vi "Read DeviceSettings.vi"(8 "error in (no error)":errorcluster, 11 "NhRegenGridSim in":refnum<class "NHRGridSim.lvclass">) -> (0 "error out":errorcluster, 2 "DeviceSettings":T1 {"Modules"."Phase (0: All)" items=["All", "A Phase", "B Phase", "C Phase"]; "Modules"."Mode" items=["3-Phase AC", "AC", "DC", "AC - AC - AC", "DC - DC - DC", "2-Phase AC - AC", "2-Phase AC - DC", "AC - AC", "AC - DC", "AC - AC - DC", "AC - DC - DC", "DC - AC", "DC - DC", "AC - DC - AC", "DC - AC - AC", "DC - AC - DC"]}, 3 "NhRegenGridSim out":refnum<class "NHRGridSim.lvclass">)   [LabVIEW 2018, in "AcPwrPlugins.lvlib" / "NHRGridSim.lvclass"]
uses:
  NHRGridSim.lvclass
  TypeDefs/Device(s)Settings_old.ctl
  TypeDefs/Modules.ctl
  NHRGridSim.lvclass/NHRGridSim.ctl
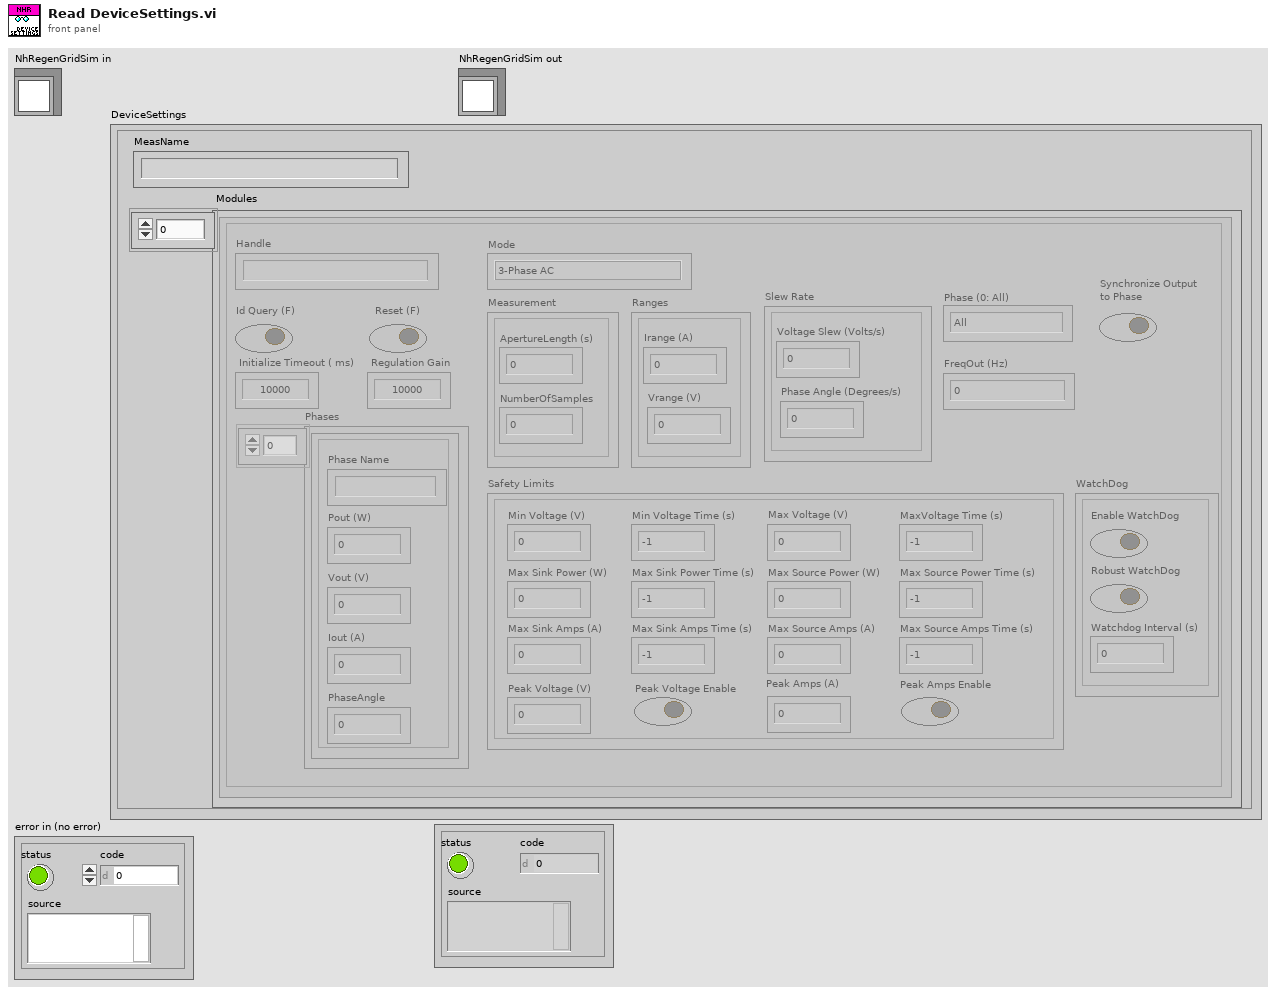
[diagram p1: front panel]
types:
  T1 = typedef "Device(s)Settings_old.ctl" = cluster{"MeasName":string, "Modules":T2}
  T2 = typedef "AcPwrPlugins.lvlib/NHRGridSim.lvclass/Modules.ctl" = cluster{"Measurement":cluster{"ApertureLength (s)":dbl, "NumberOfSamples":u32}, "Ranges":cluster{"Irange (A)":dbl, "Vrange (V)":dbl}, "Mode":u8, "Handle":string, "FreqOut (Hz)":dbl, "Connected":bool, "btnIdQuery":bool, "btnReset":bool, "Initialize Timeout ( ms)":u32, "Phase (0: All)":i32, "WatchDog":cluster{"Enable WatchDog":bool, "Robust WatchDog":bool, "Watchdog Interval (s)":dbl}, "Safety Limits":cluster{"Min Voltage (V)":dbl, "Min Voltage Time (s)":dbl, "Max Voltage (V)":dbl, "MaxVoltage Time (s)":dbl, "Max Source Amps (A)":dbl, "Max Source Amps Time (s)":dbl, "Max Sink Amps (A)":dbl, "Max Sink Amps Time (s)":dbl, "Max Source Power (W)":dbl, "Max Source Power Time (s)":dbl, "Max Sink Power (W)":dbl, "Max Sink Power Time (s)":dbl, "Peak Voltage (V)":dbl, "Peak Voltage Enable":bool, "Peak Amps (A)":dbl, "Peak Amps Enable":bool}, "Phases":cluster{"Pout (W)":dbl, "Iout (A)":dbl, "PhaseAngle":dbl, "Vout (V)":dbl, "Phase Name":string}[], "Regulation Gain":dbl, "ChangeOntheFly":bool, "Synchronize Output \nto Phase":bool, "Slew Rate":cluster{"Voltage Slew (Volts/s)":dbl, "Phase Angle (Degrees/s)":dbl}}[]
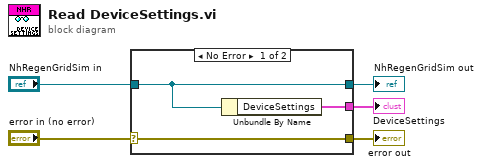
[diagram p0: block diagram]
diagram:
  n1 = case shown="No Error" "error in (no error)" {
    selector: "error in (no error)" -> [w8 w9]
    tunnel: [w8 w9] -> w4
    tunnel: [w7 w10] -> w2
    tunnel: "NhRegenGridSim in" -> [w7 w10]
    tunnel: [w6 _] -> w1
    frame No Error {
      n2 = Unbundle By Name(w7) -> ("DeviceSettings"=w6:T1)
    }
    frame Error {
    }
  }
  "error out" <- w4
  "NhRegenGridSim out" <- w2
  "DeviceSettings" <- w1
